vi "Don't Break the Finger.vi"(9 "High IR":bool, 10 "Elevator motor in":dbl, 11 "Finger Height":dbl) -> (2 "Elevator motor out":dbl)   [LabVIEW 2014]
uses:
  Robot Global Data.vi
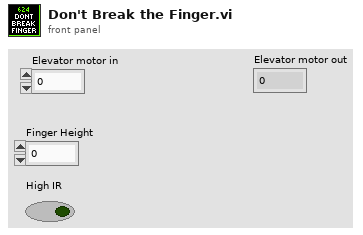
[diagram p1: front panel]
types:
  T1 = typedef "Dashboard Control Data.ctl" = cluster{"Cam Exposure":dbl, "Go to angle":dbl, "Steer PID Gains":cluster{"proportional gain (Kc)":dbl, "integral time (Ti, min)":dbl, "derivative time (Td, min)":dbl}, "Steer PID output Range":cluster{"output high":dbl, "output low":dbl}, "Pressure m \nValue":dbl, "Pressure b \nValue":dbl, "Roller Command Cluster ":T2, "Elevator":T3, "Encoder Control":T5, "Auton Settings":cluster{"Drive Dist Window Size":dbl}, "Drivetrain Settings":T6, "Lance":T7}
  T2 = typedef "Roller Control.ctl" = cluster{"Intake Speed":dbl, "Turn In Speed":dbl, "Unload Speed":dbl, "Turn Out Speed":dbl, "Ping Align Tolerance":dbl, "Tote Range Threshold":dbl, "Right Pot 0":dbl, "Pot Threshold":dbl, "Left Pot 0":dbl, "Manual 0s?":bool, "Right Pot Scale":dbl, "Left Pot Scale":dbl, "0 wait time":i32, "Zero Pots":bool, "Min Elevator Height":dbl, "Eject Time":dbl, "Eject US Threshold":dbl, "Anti-Twitch Time":u32, "Ping Caring Threshold":dbl, "Pot Diff Threshold":dbl, "Pinch Sustain":u32, "Absorb Give Up Threshold":dbl, "Untip In Threshold":dbl, "Untip Grab Range":dbl, "Ultrasonic Hold Time":u32, "Landscape Absorb Time":u32, "Pot Use Wait Time":u32, "Can Turn Stop Range":dbl, "Ignore Pressure":bool, "HP Load Speed":dbl}
  T3 = typedef "Elevator DB Control.ctl" = cluster{"PID Output Range":cluster{"output high":dbl, "output low":dbl}, "PID gains":cluster{"proportional gain (Kc)":dbl, "integral time (Ti, min)":dbl, "derivative time (Td, min)":dbl}, "Height Tolerance":sgl, " Encoder Constant":dbl, "Safe Mode Max Speed":sgl, "Eject Time":sgl, "Zeroing Speed":sgl, "Presets":T4, "Ping Detect Threshold":sgl, "Trashcan Detect Threshold":sgl, "Zero Filter Time":dbl, "Stabilizer Open Time":dbl, "Zero Creep Speed":dbl, "Max Current":dbl, "Current Trip Time":dbl, "Abort Pitch":dbl, "Finger m":dbl, "Finger b":dbl, "Finger max ":dbl, "Finger Stabilizer":dbl, "Finger Store":dbl, "Finger Stop Store":dbl, "Stabilizer Close Time":dbl, "HP Finger Store":dbl, "HP Finger Stop Store":dbl, "Finger min":dbl, "Unstick gain":dbl, "Roller Wait":dbl}
  T4 = typedef "Elevator Presets.ctl" = cluster{"Pickup 2 w/ Tote":sgl, "Pickup 2 w/ Trashcan":sgl, "Pickup 3 w/ Tote":sgl, "Pickup 3 w/ Trashcan":sgl, "Bottom":sgl, "Pickup 1 w/ Tote":sgl, "Pickup Trashcan":sgl, "Pickup 1 w/ Trashcan":sgl, "Eject":sgl, "Hold Low":sgl, "Step add height":sgl, "Untip Lift":dbl, "Drop Stack":dbl, "HP Load Hold":dbl, "HP Load Drop":dbl, "HP Load Finger":dbl, "HP Load Hold Can":dbl, "Store can max":dbl, "HP Drag Score":dbl, "HP Store can max":dbl, "HP Drag Finish":dbl, "HP Carry min":dbl, "HP Finger Anti-Crash":dbl, "Finger trashcan avoid":dbl}
  T5 = typedef "Encoder Control.ctl" = cluster{"Left Tick Constant":dbl, "Right Tick Constant":dbl, "Center Tick Constant":dbl, "Reset?":bool, "Y Dist":cluster{"PID gains":cluster{"proportional gain (Kc)":dbl, "integral time (Ti, min)":dbl, "derivative time (Td, min)":dbl}}, "X Dist":cluster{"PID gains":cluster{"proportional gain (Kc)":dbl, "integral time (Ti, min)":dbl, "derivative time (Td, min)":dbl}}, "Y Stop Thresh":dbl, "Y Stop Speed":dbl, "X Stop Thresh":dbl, "X Stop Speed":dbl}
  T6 = typedef "Drivetrain Settings.ctl" = cluster{"Gyro Tolerance":sgl, "Strafe Correct max steer":sgl, "Strafe Timer Wait":sgl, "Throttle Ramp (ms)":sgl, "Strafe Ramp (ms)":sgl, "Angular rate compensation":bool, "Throttle to Rate Scale":sgl, "Rate compensation gain":sgl, "Creep Steer":sgl, "Creep Throttle":sgl}
  T7 = typedef "Pike DB Controls.ctl" = cluster{"Down Speed":dbl, "Up Speed":dbl, "Max Down Time":dbl, "Max Up Time":dbl, "Current Limit":dbl}
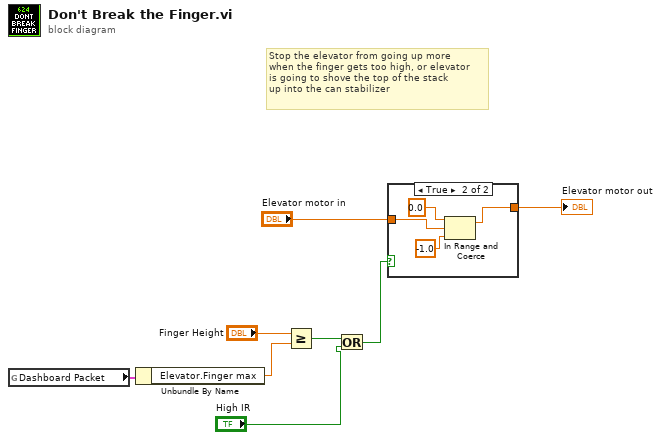
[diagram p0: block diagram]
diagram:
  # "Stop the elevator from going up more\nwhen the finger gets too high, or elevator\nis going to shove the top of the stack\nup into the can stabilizer"
  n1 = global read "Robot Global Data.vi" "Dashboard Packet"() -> (w5:T1)
  n2 = Unbundle By Name(w5) -> ("Elevator.Finger max"=w4:dbl)
  n3 = Greater Or Equal?(x="Finger Height", y=w4) -> (x >= y?=w3:bool)
  n4 = Or(x=w3, y="High IR") -> (x .or. y?=w2:bool)
  n5 = case shown="True" w2 {
    tunnel: "Elevator motor in" -> [w9 w13]
    tunnel: [w9 w10] -> w7
    frame False {
    }
    frame True {
      n6 = In Range and Coerce(upper limit=0.0, x=w13, lower limit=-1.0) -> (coerced(x)=w10:dbl)  [unwired: 1 out]
    }
  }
  "Elevator motor out" <- w7
